vi "Valid Self Defined Pattern Index or Not.vi"(8 "error in (no error)":errorcluster, 11 "customized character code":u8) -> (0 "error out":errorcluster)   [LabVIEW 2017, in "HD44780.lvclass"]
uses:
  HD44780.lvclass
  Common/HD44780 Common.lvlib
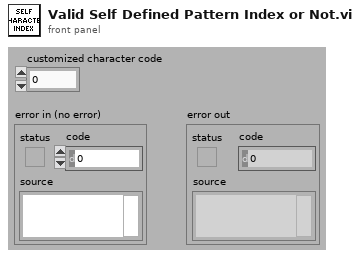
[diagram p1: front panel]
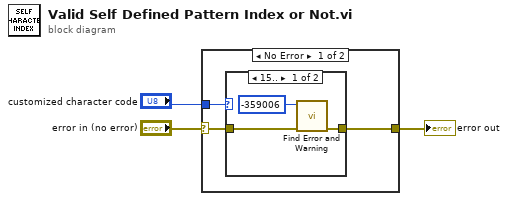
[diagram p0: block diagram]
diagram:
  n1 = case shown="No Error" "error in (no error)" {
    selector: "error in (no error)" -> [w5 w11]
    tunnel: [w6 w11] -> w2
    tunnel: "customized character code" -> [w4 _]
    frame No Error {
      n2 = case shown="15.." w4 {
        tunnel: [w9 w10] -> w6
        tunnel: w5 -> [w7 w10]
        frame 15.. {
          n3 = call "Find Error and Warning.vi"("error in (no error)"=w7, "error code"=-359006) -> ("error out"=w9:errorcluster)  [unwired: 9 in]
        }
        frame 1, Default {
        }
      }
    }
    frame Error {
    }
  }
  "error out" <- w2
